vi "Server Properties.vi"(8 "error in (no error)":errorcluster, 11 ".NET Refnum in":refnum<k24>) -> (0 "error out":errorcluster, 2 "Cluster":T1, 3 ".NET Refnum out":refnum<k24>)   [LabVIEW 2024, in "LV_OPC_NET.lvlib"]
uses:
  LV_OPC_NET.lvlib
  C:/Users/108003658/OneDrive - Baker Hughes/Desktop/LV_OPC-Client-x64/LV_OPC_Test/OPC.NET/OpcNetApi.dll
  OpcNetApi.dll
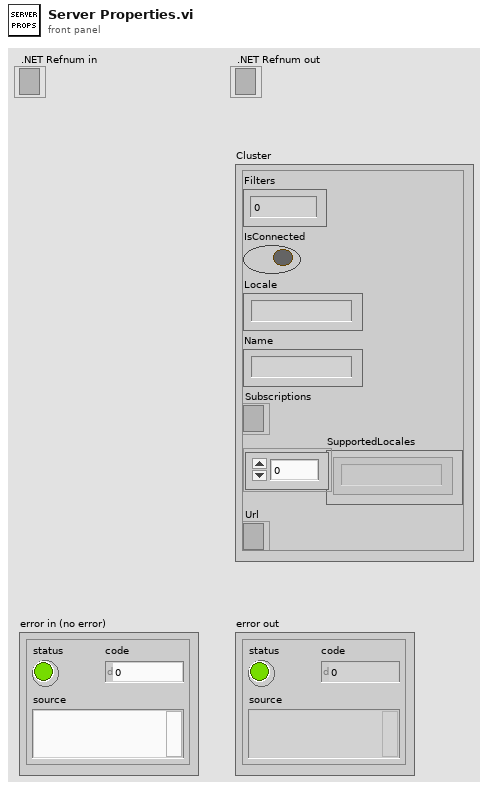
[diagram p1: front panel]
types:
  T1 = cluster{"Filters":i32, "IsConnected":bool, "Locale":string, "Name":string, "Subscriptions":refnum<k24>, "SupportedLocales":string[], "Url":refnum<k24>}
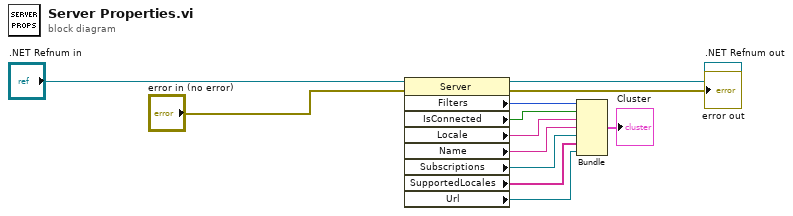
[diagram p0: block diagram]
diagram:
  n1 = property class="Server"(reference=".NET Refnum in", error in="error in (no error)") -> (reference out=→".NET Refnum out":refnum<k24>, error out=→"error out":errorcluster, "Filters"=w2:i32, "IsConnected"=w3:bool, "Locale"=w4:string, "Name"=w5:string, "Subscriptions"=w6:refnum<k24>, "SupportedLocales"=w7:string[], "Url"=w8:refnum<k24>)
  n2 = Bundle("Filters"=w2, "IsConnected"=w3, "Locale"=w4, "Name"=w5, "Subscriptions"=w6, "SupportedLocales"=w7, "Url"=w8) -> (→"Cluster":T1)  [unwired: 1 in]
